vi "Gazebo_TopicInit.vi"(9 "Action":T1=enum."Subscriber", 10 "Message Type":string, 11 "Topic":string(combo)="/clock") -> (3 "ROS out":T2)   [LabVIEW 2012]
doc: "Initializes the specified topic. Topics listed in the drop down menu will automatically populate the message type. If you enter a topic not included in the drop down list, remember to specify the message type."
uses:
  <userlib>/ROSforLV/ROS/Code/SubVIs/_ROSControl.ctl
  <userlib>/ROSforLV/ROS/Code/SubVIs/_ROSDirection.ctl
panel:
  # "running an empty world with \"rosrun gazebo_ros gazebo\" \nand then \"rostopic list\" shows the following active topics:\n\n/clock\n/gazebo/link_states\n/gazebo/model_states\n/gazebo/parameter_descriptions\n/gazebo/parameter_updates\n/gazebo/set_link_state\n/gazebo/set_model_state\n/rosout\n/rosout_agg"
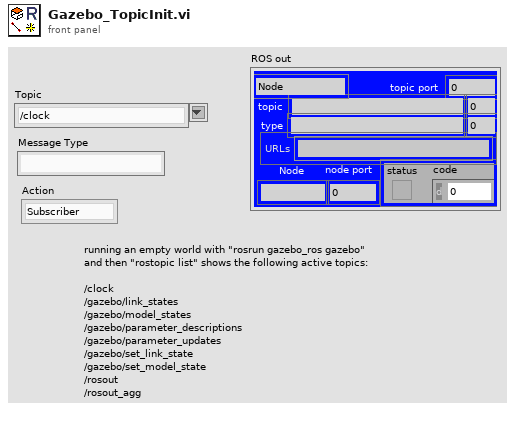
[diagram p1: front panel]
types:
  T1 = typedef "_ROSDirection.ctl" = enum16{"Node", "Publisher", "Subscriber", "Service Client"}
  T2 = typedef "_ROSControl.ctl" = cluster{"topic port":u16, "Node":string, "topic":string, "type":string, "node port":u32, "error ":errorcluster, "Direction":T1, "APIs":string[], "Update (ms)":u16, "write queue":u16}
  T3 = cluster{"Topic":string, "Type":string, "Action":T1, "Update (ms)":u16, "write queue":u16}
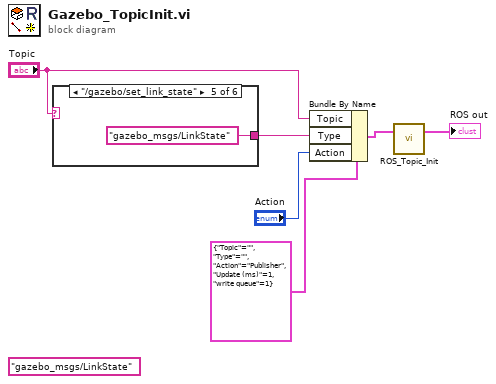
[diagram p0: block diagram]
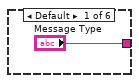
[diagram p2: hidden frame]
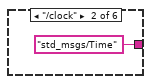
[diagram p3: hidden frame]
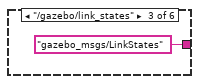
[diagram p4: hidden frame]
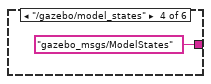
[diagram p5: hidden frame]
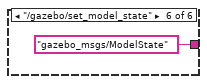
[diagram p6: hidden frame]
diagram:
  (unwired) "gazebo_msgs/LinkState" ("Topic")
  n1 = case shown="\"/gazebo/set_link_state\"" "Topic" {
    tunnel: ["Message Type" "std_msgs/Time" ("Topic") "gazebo_msgs/LinkStates" ("Topic") "gazebo_msgs/ModelStates" ("Topic") "gazebo_msgs/LinkState" ("Topic") "gazebo_msgs/ModelState" ("Topic")] -> w2
    frame Default {
    }
    frame "/clock" {
    }
    frame "/gazebo/link_states" {
    }
    frame "/gazebo/model_states" {
    }
    frame "/gazebo/set_link_state" {
    }
    frame "/gazebo/set_model_state" {
    }
  }
  n2 = Bundle By Name(cluster=T3 {"Topic"="", "Type"="", "Action"=enum."Publisher", "Update (ms)"=1, "write queue"=1} ("Definitions"), "Topic"="Topic", "Type"=w2, "Action"="Action") -> (w1:T3)
  n3 = call <userlib>:"ROS_Topic_Init.vi"("Definitions"=w1) -> ("ROS out"=→"ROS out":T2)  [unwired: 2 in]
